vi "ReadError.vi"() -> ()   [LabVIEW 2014, in "YbTempCtrl.lvlib"]
uses:
  YbTempCtrl.lvlib
panel:
  in  "Input channel":enum16{"1T", "1V", "2T", "2V"}(ring)
  in  "Wait time / ms":u32
  in  "stop":bool
  in  "VISA resource name":refnum<visa-resource-name>="COM4"
  out "Error":dbl(graph)
  # "Error signal monitor"
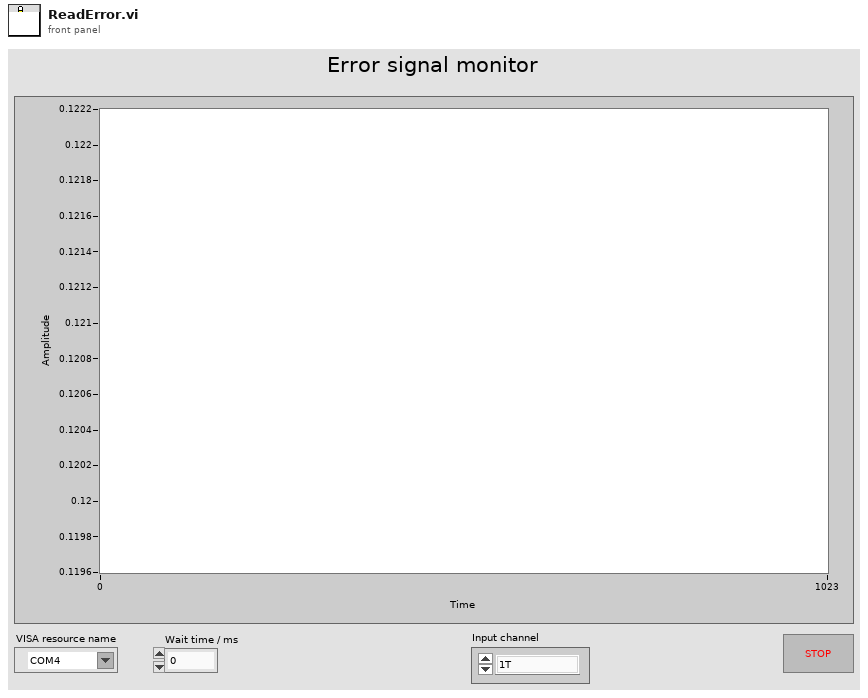
[diagram p1: front panel]
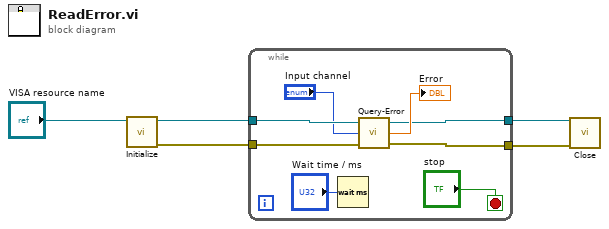
[diagram p0: block diagram]
diagram:
  n1 = call "Initialize.vi"("VISA resource name"="VISA resource name") -> ("error out"=w3:errorcluster, "VISA resource name out"=w4:refnum<visa-resource-name>)  [unwired: 9 in]
  n2 = while {
    tunnel: w4 -> [w12]
    tunnel: w3 -> [w11]
    tunnel: [w8] -> w1
    tunnel: [w7] -> w2
    stop <- "stop" stop-if-true
    n3 = Wait (ms)(milliseconds to wait="Wait time / ms") -> ()  [unwired: 1 out]
    n4 = call "Query-Error.vi"("error in (no error)"=w11, "Input channel"="Input channel", "VISA resource name"=w12) -> ("error out"=w7:errorcluster, "Error Signal / V"=→"Error":dbl, "VISA resource name out"=w8:refnum<visa-resource-name>)
  }
  n5 = call "Close.vi"("error in (no error)"=w2, "VISA resource name"=w1) -> ()  [unwired: 9 in, 1 out]
